vi "Calibration_Analysis.vi"(2 "Root Name":string[](array[string]), 3 "New Calib Filenames":path[](array[path]), 4 "Instrument type":T1=enum."Hot wire", 5 "Clear Calib History":bool) -> (0 "Error String":string, 1 "Max % Error":dbl format="%.2f")   [LabVIEW 2010]
uses:
  Controls/Cal_Inst_type.ctl
  Globals/Preference_global.vi
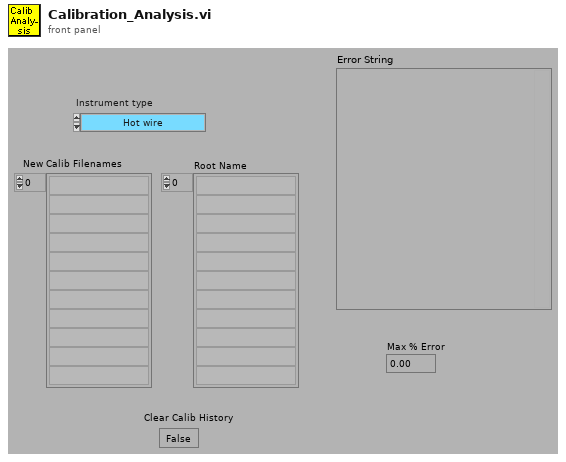
[diagram p1: front panel]
types:
  T1 = typedef "Cal_Inst_type.ctl" = enum16{"Propeller anemometer", "Pressure Transducer", "Hot wire", "Cross wire velocity", "Cross wire angle", "Generic Linear", "Generic Polynomial", "Generic BackPoly", "Fast FID", "Thermocouple", "Cold wire", "Pulsed Wire"}
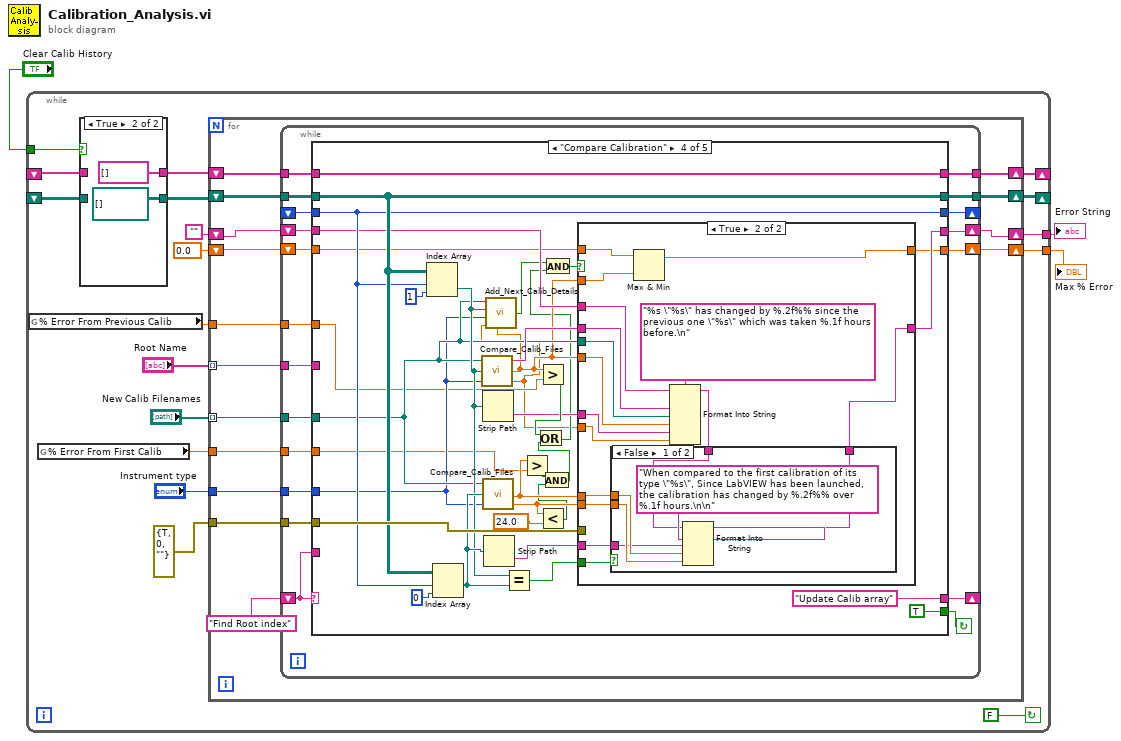
[diagram p0: block diagram]
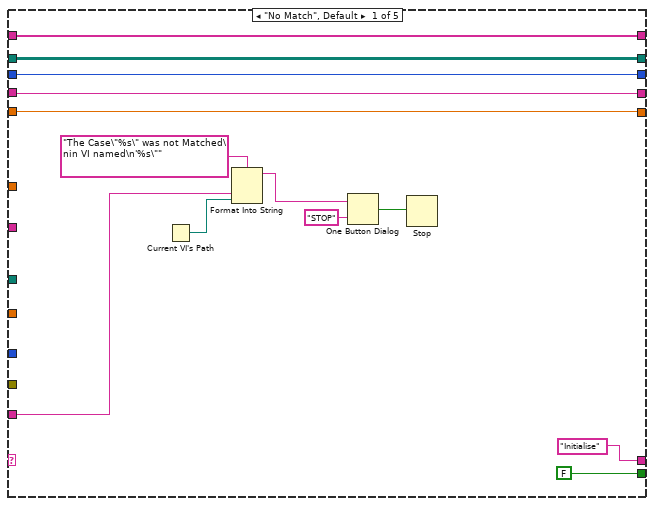
[diagram p3: hidden frame]
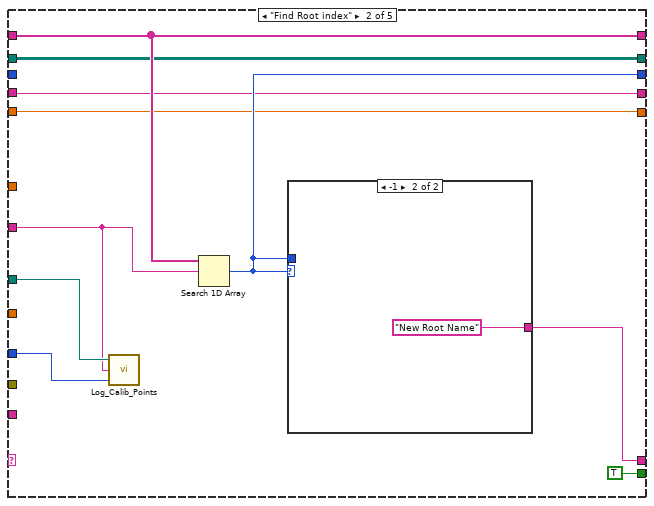
[diagram p4: hidden frame]
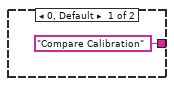
[diagram p5: hidden frame]
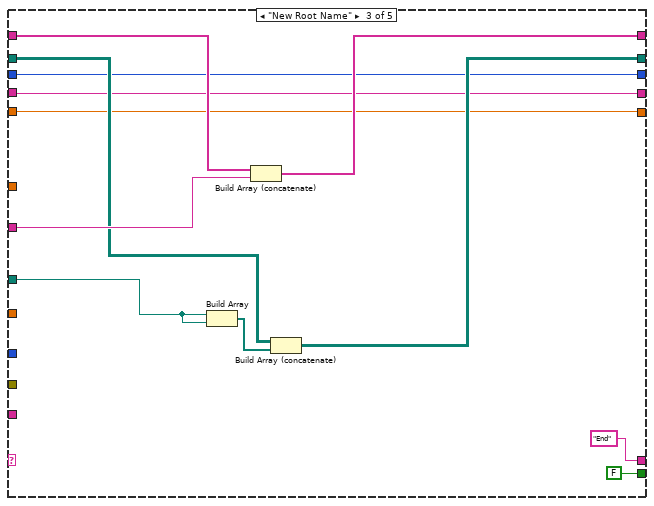
[diagram p6: hidden frame]
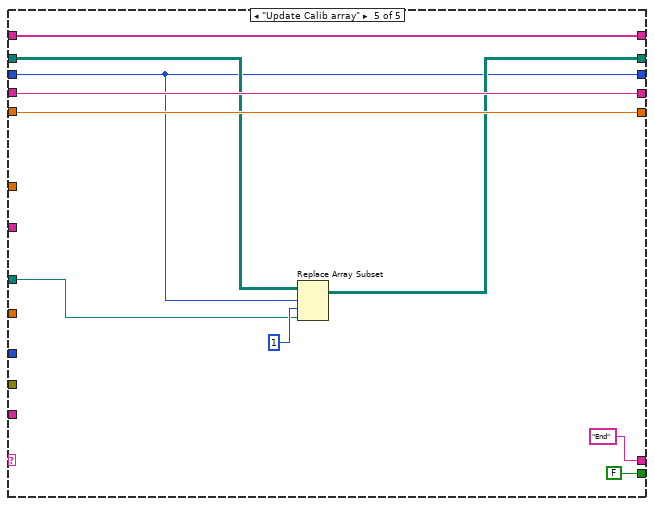
[diagram p9: hidden frame]
diagram:
  n1 = while {
    tunnel: "Clear Calib History" -> [w11]
    tunnel: [w13] -> w2
    tunnel: [w14] -> w3
    shift-left: _ -> [w7]
    shift-right: [w20] -> _
    shift-left: _ -> [w10]
    shift-right: [w21] -> _
    stop <- FALSE continue-if-true
    n2 = global read "Preference_global.vi" "% Error From Previous Calib"() -> (w6:dbl)
    n3 = global read "Preference_global.vi" "% Error From First Calib"() -> (w5:dbl)
    n4 = case shown="True" w11 {
      tunnel: w10 -> [w23 _]
      tunnel: [w23 string[] []] -> w9
      tunnel: [w22 path[][] []] -> w8
      tunnel: w7 -> [w22 _]
      frame False {
      }
      frame True {
      }
    }
    n5 = for {
      shift-right: [w39] -> w21
      shift-left: w9 -> [w38]
      shift-right: [w37] -> w20
      shift-left: w8 -> [w36]
      tunnel: "Root Name" -> [w35] mode=indexing
      tunnel: "New Calib Filenames" -> [w34] mode=indexing
      tunnel: "Instrument type" -> [w33]
      tunnel: errorcluster {"status"=TRUE, "code"=0, "source"=""} ("error in (no error)") -> [w32]
      shift-right: [w30] -> w14
      shift-left: "" -> [w31]
      shift-right: [w28] -> w13
      shift-left: 0.0 -> [w29]
      tunnel: w6 -> [w27]
      tunnel: w5 -> [w26]
      n6 = while {
        tunnel: w26 -> [w41]
        tunnel: w27 -> [w42]
        shift-left: w29 -> [w43]
        shift-right: [w44] -> w28
        shift-left: w31 -> [w46]
        shift-right: [w45] -> w30
        tunnel: w32 -> [w47]
        tunnel: w33 -> [w48]
        tunnel: w34 -> [w49]
        tunnel: w35 -> [w51]
        shift-left: _ -> [w50]
        shift-right: [w52] -> _
        tunnel: w36 -> [w53]
        tunnel: [w54] -> w37
        tunnel: w38 -> [w55]
        tunnel: [w56] -> w39
        shift-left: "Find Root index" -> [w57]
        shift-right: [w58] -> _
        stop <- w59 continue-if-true
        n7 = case shown="\"Compare Calibration\"" w57 {
          tunnel: [FALSE TRUE FALSE TRUE FALSE] -> w59
          tunnel: ["Initialise" w80 "End" "Update Calib array" "End"] -> w58
          tunnel: w57 -> [w67 _ _ _ _]
          tunnel: [w64 w81 w93 w130 w165] -> w56
          tunnel: w55 -> [w64 w81 w95 w130 w165]
          tunnel: [w63 w78 w90 w124 w160] -> w54
          tunnel: w53 -> [w63 w78 w91 w124 w158]
          tunnel: [w62 w79 w89 w123 w157] -> w52
          tunnel: w51 -> [_ w74 w94 _ _]
          tunnel: w50 -> [w62 _ w89 w123 w157]
          tunnel: w49 -> [_ w75 w92 w110 w156]
          tunnel: w48 -> [_ w73 _ w109 _]
          tunnel: w47 -> [_ _ _ w127 _]
          tunnel: w46 -> [w61 w77 w86 w121 w164]
          tunnel: [w61 w77 w86 w122 w164] -> w45
          tunnel: [w60 w76 w85 w116 w163] -> w44
          tunnel: w43 -> [w60 w76 w85 w115 w163]
          tunnel: w42 -> [_ _ _ w107 _]
          tunnel: w41 -> [_ _ _ w106 _]
          frame "No Match", Default {
            n8 = Current VI's Path() -> (path=w66:path)
            n9 = Format Into String(format string="The Case\"%s\" was not Matched\nin VI named\n'%s\"" ("Format String"), w67, w66) -> (resulting string=w70:string)  [unwired: 2 in, 1 out]
            n10 = One Button Dialog(message=w70, button name ("OK")="STOP") -> (true=w68:bool)
            n11 = Stop(stop? (T)=w68) -> ()
          }
          frame "Find Root index" {
            n12 = call "Log_Calib_Points.vi"("Instrument type"=w73, "Root name"=w74, "Calib file"=w75) -> ()  [unwired: 3 out]
            n13 = Search 1D Array(1D array=w81, element=w74) -> (index of element=w79:i32)  [unwired: 1 out]
            n14 = case shown="-1" w79 {
              tunnel: ["Compare Calibration" "New Root Name"] -> w80
              tunnel: w79 -> [_ _]
              frame 0, Default {
              }
              frame -1 {
              }
            }
          }
          frame "New Root Name" {
            n15 = Build Array(w92, w92) -> (w96:path[])
            n16 = Build Array (concatenate)(w95, w94) -> (w93:string[])
            n17 = Build Array (concatenate)(w91, w96) -> (w90:path[][])
          }
          frame "Compare Calibration" {
            n18 = Index Array(array=w124, index (row)=w123, index (col)=1 ("Index")) -> (element=w111:path)
            n19 = Index Array(array=w124, index (row)=w123, index (col)=0 ("Index")) -> (element=w113:path)
            n20 = call "Compare_Calib_Files.vi"("Instrument type"=w109, "Calib file Orig"=w111, "Calib file New"=w110) -> ("Calib Time Separation (Hours)"=w97:dbl, "% Change"=w108:dbl, "Calib name"=w126:string)
            n21 = Strip Path(path=w111) -> (name=w114:string)  [unwired: 1 out]
            n22 = call "Compare_Calib_Files.vi"("Instrument type"=w109, "Calib file Orig"=w113, "Calib file New"=w110) -> ("Calib Time Separation (Hours)"=w102:dbl, "% Change"=w118:dbl)  [unwired: 1 out]
            n23 = Strip Path(path=w113) -> (name=w112:string)  [unwired: 1 out]
            n24 = call "Add_Next_Calib_Details.vi"("% Change"=w108, "Hours between calibrations"=w97, "Instrument type"=w109, "Calib file Orig"=w111, "Calib file New"=w110) -> ("Results Files Updated"=w105:bool)  [unwired: 1 out]
            n25 = Equal?(x=w111, y=w113) -> (x = y?=w119:bool)
            n26 = Greater?(x=w118, y=w106) -> (0:w100:bool)
            n27 = Greater?(x=w108, y=w107) -> (0:w117:bool)
            n28 = Less?(x=w102, y=24.0) -> (x < y?=w99:bool)
            n29 = And(x=w100, y=w99) -> (x .and. y?=w98:bool)
            n30 = Or(x=w117, y=w98) -> (x .or. y?=w104:bool)
            n31 = And(x=w105, y=w104) -> (x .and. y?=w103:bool)
            n32 = case shown="True" w103 {
              tunnel: w127 -> [_ _]
              tunnel: w97 -> [_ w138]
              tunnel: w108 -> [_ w145]
              tunnel: w126 -> [_ w147]
              tunnel: w110 -> [_ w146]
              tunnel: w118 -> [_ w142]
              tunnel: w102 -> [_ w141]
              tunnel: w121 -> [w132 w144]
              tunnel: [w132 w139] -> w122
              tunnel: w119 -> [_ w143]
              tunnel: w108 -> [_ w135]
              tunnel: [w131 w133] -> w116
              tunnel: w115 -> [w131 w134]
              tunnel: w114 -> [_ w137]
              tunnel: w112 -> [_ w136]
              frame False {
              }
              frame True {
                n33 = Max & Min(x=w134, y=w135) -> (max(x,y)=w133:dbl)  [unwired: 1 out]
                n34 = Format Into String(format string="%s \"%s\" has changed by %.2f%% since the previous one \"%s\" which was taken %.1f hours before.\n" ("Format String"), initial string=w144, w147, w146, w145, w137, w138) -> (resulting string=w140:string)  [unwired: 1 in, 1 out]
                n35 = case shown="False" w143 {
                  tunnel: w142 -> [w153 _]
                  tunnel: w141 -> [w152 _]
                  tunnel: w140 -> [w151 w155]
                  tunnel: [w150 w155] -> w139
                  tunnel: w136 -> [w149 _]
                  frame False {
                    n36 = Format Into String(format string="When compared to the first calibration of its type \"%s\", Since LabVIEW has been launched, the calibration has changed by %.2f%% over %.1f hours.\n\n" ("Format String"), initial string=w151, w149, w153, w152) -> (resulting string=w150:string)  [unwired: 1 in, 1 out]
                  }
                  frame True {
                  }
                }
              }
            }
          }
          frame "Update Calib array" {
            n37 = Replace Array Subset(array=w158, new element=w156, index (row)=w157, index (col)=1 ("Index")) -> (w160:path[][])
          }
        }
      }
    }
  }
  "Error String" <- w3
  "Max % Error" <- w2
